vi "SuperVI.vi"() -> ()   [LabVIEW 2021]
uses:
  <vilib>/MakerHub/LINX/Public/Peripherals/Digital/Digital Write 1 Chan.vi
  <vilib>/MakerHub/LINX/Public/Peripherals/Digital/Digital Write N Chans.vi
  <vilib>/MakerHub/LINX/Private/Local IO/LinxDigitalWrite.vi
  <vilib>/MakerHub/LINX/Public/Utilities/Check Channel.vi
  <vilib>/MakerHub/LINX/Public/Utilities/Open Serial.vi
  <vilib>/MakerHub/LINX/Private/Utilties/Generate Error.vi
  <vilib>/MakerHub/LINX/LMH-LINX.lvlib
panel:
  out "Adjusted motor steps":i32
  out "Single Plot":dbl[](graph)
  in  "Motor steps":i32
  in  "Serial Port":refnum<visa-resource-name>="N/A"
  out "error out":errorcluster
  in  "error in (no error)":errorcluster
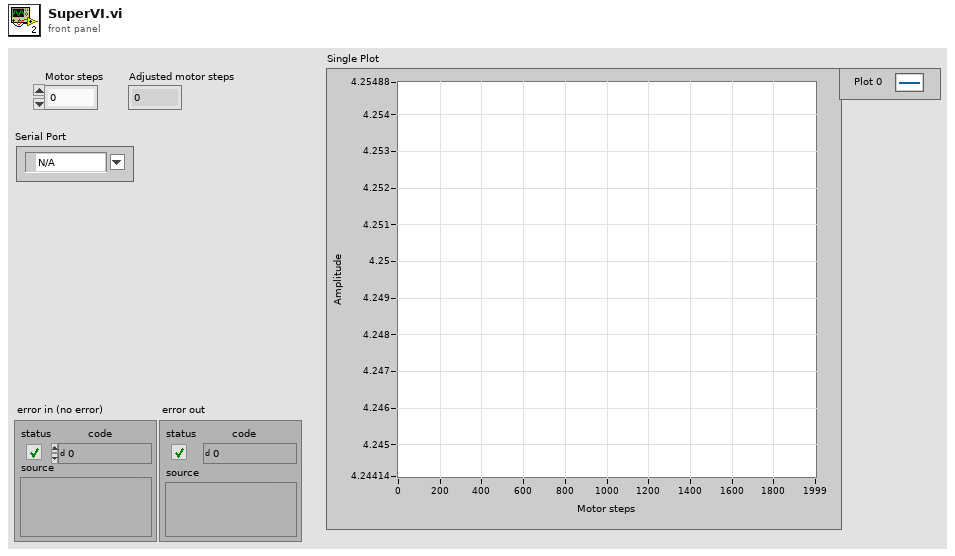
[diagram p1: front panel]
types:
  T1 = typedef "LMH-LINX.lvlib/LINX Ref.ctl" = cluster{"IO":T2, "Interface":T3, "LINX Device Config":T4}
  T2 = typedef "LMH-LINX.lvlib/Platform.ctl" = enum16{"Remote", "Local"}
  T3 = typedef "LMH-LINX.lvlib/Interface.ctl" = enum16{"Serial", "TCP"}
  T4 = typedef "LMH-LINX.lvlib/Device.lvlib/LINX Device Config.ctl" = cluster{"Interface":T3, "COM Port":refnum<visa-resource-name>, "TCP Configuration":T5, "Device Family":u8, "Device ID":u8, "Device Name":string, "TCP Ref":refnum<k5>, "Channels":T6}
  T5 = typedef "LMH-LINX.lvlib/Device.lvlib/TCP Config.ctl" = cluster{"IP Address":string, "Port":u16}
  T6 = typedef "LMH-LINX.lvlib/Channels.ctl" = cluster{"DI":u8[], "DO":u8[], "AI":u8[], "AO":u8[], "PWM":u8[], "QE":u8[], "UART":u8[], "I2C 2":u8[], "SPI":u8[], "CAN":u8[], "Servo":u8[], "AI Ref (V)":dbl, "AI Resolution (Bits)":u8, "AO Ref (V)":dbl, "AO Resolution (Bits)":u8}
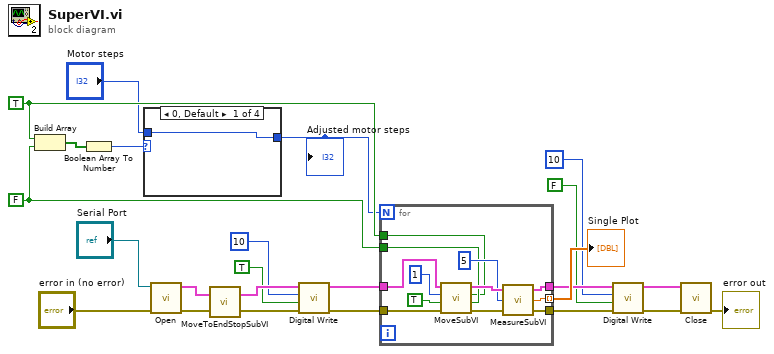
[diagram p0: block diagram]
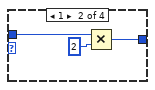
[diagram p2: hidden frame]
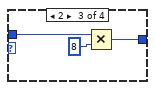
[diagram p3: hidden frame]
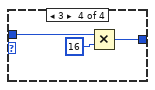
[diagram p4: hidden frame]
diagram:
  w5 = FALSE ("M1")
  w6 = TRUE ("M0")
  n1 = Build Array(w6, w5) -> (w4:bool[])
  n2 = Boolean Array To Number(Boolean array=w4) -> (number=w3:u32)
  n3 = case shown="0, Default" w3 {
    tunnel: "Motor steps" -> [w25 w28 w30 w34]
    tunnel: [w25 w27 w31 w33] -> w1
    frame 0, Default {
    }
    frame 1 {
      n4 = Multiply(x=w28, y=2) -> (x*y=w27:i32)
    }
    frame 2 {
      n5 = Multiply(x=w30, y=8) -> (x*y=w31:i32)
    }
    frame 3 {
      n6 = Multiply(x=w34, y=16) -> (x*y=w33:i32)
    }
  }
  "Adjusted motor steps" <- w1
  n7 = call-poly <vilib>:"Open.vi"("Error In"="error in (no error)", "Serial Port"="Serial Port") -> ("Error Out"=w22:errorcluster, "LINX Resource"=w21:T1)  [unwired: 7 in, 1 out]
  n8 = call "MoveToEndStopSubVI.vi"("error in (no error)"=w22, "LINX Resource"=w21) -> ("error out"=w11:errorcluster, "LINX Resource 2"=w18:T1)
  n9 = call-poly <vilib>:"Digital Write.vi"("Error In"=w11, "Output Value"=TRUE, "DO Channel"=u8 10, "LINX Resource"=w18) -> ("Error Out"=w12:errorcluster, "LINX Resource"=w17:T1)  [unwired: 6 in]
  n10 = for {
    N: w1 -> [_]
    tunnel: [w41] -> w19 mode=indexing
    tunnel: [w40] -> w16
    tunnel: [w39] -> w13
    tunnel: w17 -> [w38]
    tunnel: w12 -> [w37]
    tunnel: w5 -> [w36]
    tunnel: w6 -> [w35]
    n11 = call "MoveSubVI.vi"("M1"=w36, "M0"=w35, "error in (no error)"=w37, "Direction"=TRUE, "Number of Steps"=u32 1, "LINX Resource"=w38) -> ("error out"=w45:errorcluster, "LINX Resource 2"=w46:T1)
    n12 = call "MeasureSubVI.vi"("error in (no error)"=w45, "Number of Samples"=5, "LINX Resource"=w46) -> ("error out"=w39:errorcluster, "Average"=w41:dbl, "LINX Resource 2"=w40:T1)
  }
  "Single Plot" <- w19
  n13 = call-poly <vilib>:"Digital Write.vi"("Error In"=w13, "Output Value"=FALSE, "DO Channel"=u8 10, "LINX Resource"=w16) -> ("Error Out"=w14:errorcluster, "LINX Resource"=w15:T1)  [unwired: 6 in]
  n14 = call <vilib>:"Close.vi"("Error In"=w14, "LINX Resource"=w15) -> ("Error Out"=→"error out":errorcluster)  [unwired: 9 in]
